vi "Obtener_Posiciones_En_Blanco.vi"(1 "Numero_Columnas":dbl, 2 "Numero_Filas":dbl, 3 "Pistas":T1(array[cluster]), 4 "Posiciones_Minas":string[](array[string])) -> (0 "Posiciones_En_Blanco":string[](array[string]))   [LabVIEW 2019]
doc: "Retorna todas las posiciones que no estan asociadas a una mina o a una pista.\nRetorna una lista de posiciones tipo String con formato 'x,y'."
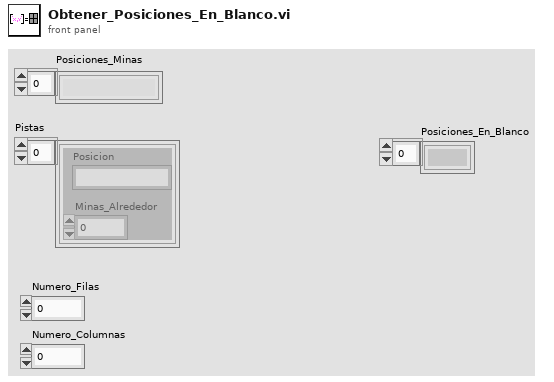
[diagram p1: front panel]
types:
  T1 = cluster{"Posicion":string, "Minas_Alrededor":dbl}[]
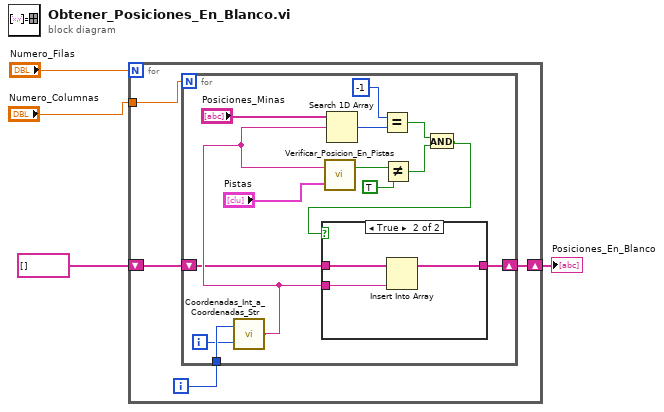
[diagram p0: block diagram]
diagram:
  n1 = for {
    N: "Numero_Filas" -> [_]
    tunnel: "Numero_Columnas" -> [w8]
    shift-right: [w6] -> w1
    shift-left: string[] [] -> [w5]
    i -> [w7]
    n2 = for {
      N: w8 -> [_]
      tunnel: w7 -> [w22]
      shift-right: [w10] -> w6
      shift-left: w5 -> [w9]
      i -> [w21]
      n3 = call "Coordenadas_Int_a_Coordenadas_Str.vi"("Columna"=w21, "Fila"=w22) -> ("Posicion_str"=w11:string)
      n4 = call "Verificar_Posicion_En_Pistas.vi"("Pistas"="Pistas", "Posicion"=w11) -> ("Es_Una_Pista"=w16:bool)  [unwired: 1 out]
      n5 = Search 1D Array(1D array="Posiciones_Minas", element=w11) -> (index of element=w19:i32)  [unwired: 1 in]
      n6 = Equal?(x=-1, y=w19) -> (x = y?=w14:bool)
      n7 = Not Equal?(x=w16, y=TRUE) -> (x != y?=w13:bool)
      n8 = And(x=w14, y=w13) -> (x .and. y?=w12:bool)
      n9 = case shown="True" w12 {
        tunnel: w11 -> [_ w26]
        tunnel: [w23 w25] -> w10
        tunnel: w9 -> [w23 w24]
        frame False {
        }
        frame True {
          n10 = Insert Into Array(array=w24, new element=w26) -> (w25:string[])  [unwired: 1 in]
        }
      }
    }
  }
  "Posiciones_En_Blanco" <- w1
